vi "Set Wavelength.vi"(8 "error in":errorcluster, 9 "Interaction Type":string, 10 "Wavelength":dbl, 11 "reference":refnum<k24>) -> (0 "error out":errorcluster, 3 "reference out":refnum<k24>)   [LabVIEW 2020, in "Topas4.lvlib"]
uses:
  Topas4.lvlib
  C:/Windows/SysWOW64/Topas4Lib.dll
  Windows/SysWOW64/Topas4Lib.dll
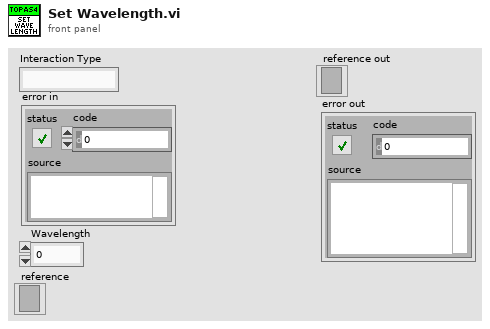
[diagram p1: front panel]
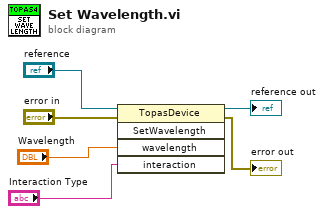
[diagram p0: block diagram]
diagram:
  n1 = invoke class="TopasDevice" method="SetWavelength"(reference="reference", error in="error in", "wavelength"="Wavelength", "interaction"="Interaction Type") -> (reference out=→"reference out":refnum<k24>, error out=→"error out":errorcluster)  [unwired: 1 in, 3 out]
